vi "main.vi"() -> ()   [LabVIEW 2011]
panel:
  out "Table Control":string[][](table)
  in  "Run Tests":bool
  out "2D Picture":picture
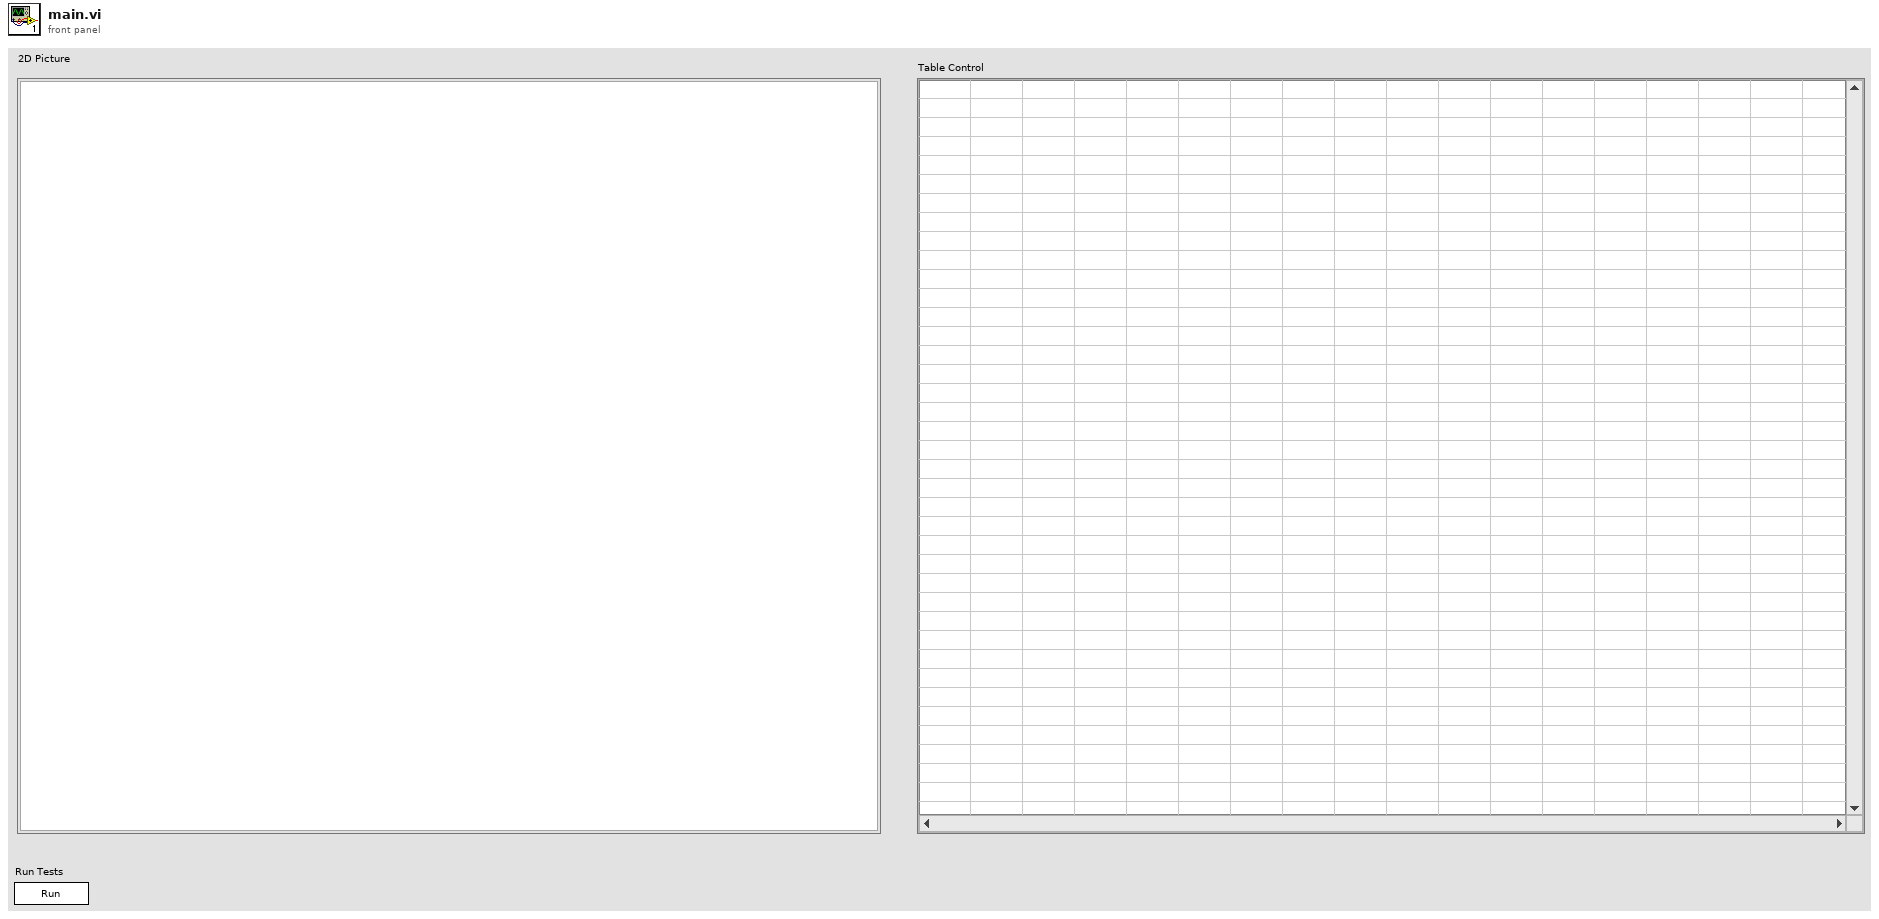
[diagram p1: front panel]
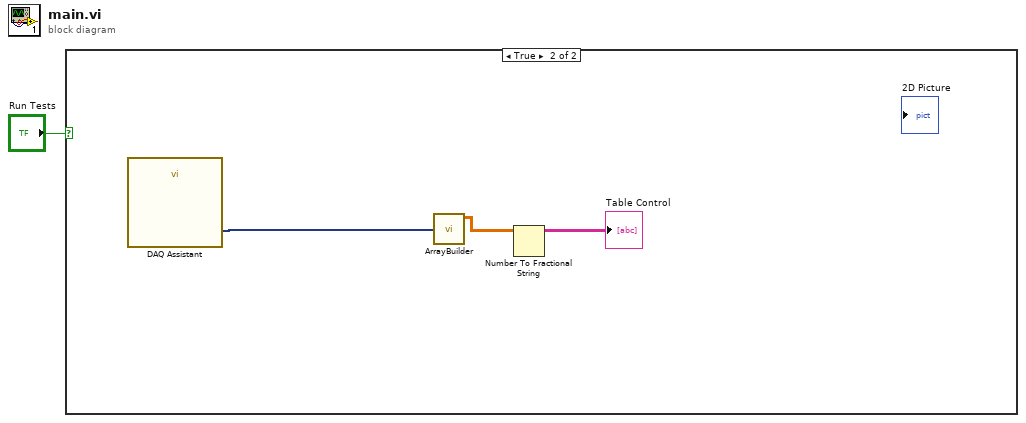
[diagram p0: block diagram]
diagram:
  n1 = case shown="True" "Run Tests" {
    frame False {
    }
    frame True {
      n2 = call "DAQ Assistant"() -> ("data"=w4:dynamicdata)  [unwired: 17 in, 2 out]
      n3 = call "ArrayBuilder.vi"("data"=w4) -> ("Array"=w3:dbl[][])  [unwired: 10 in]
      n4 = Number To Fractional String(number=w3) -> (F-format string=→"Table Control":string[][])  [unwired: 3 in]
    }
  }
